vi "ConfigDevice.vi"(8 "error in (no error)":errorcluster, 11 "NhRegenGridSim in":refnum<class "NHRGridSim.lvclass">) -> (0 "error out":errorcluster, 3 "NhRegenGridSim out":refnum<class "NHRGridSim.lvclass">)   [LabVIEW 2018, in "AcPwrPlugins.lvlib" / "NHRGridSim.lvclass"]
doc: "This VI configures the instrument for the properties set such as instrument mode, slew, power level, etc."
uses:
  NHRGridSim.lvclass
  TypeDefs/ConfigDevicesTypeDef.ctl
  <instrlib>/NH Research 9400 Series/Public/Utility/Query Capabilities (Aperture).vi
  <vilib>/Utility/error.llb/Error Cluster From Error Code.vi
  <vilib>/ErrorRing/Error Ring.xnode
  <instrlib>/NH Research 9400 Series/NH Research 9400 Series.lvlib
  TypeDefs/RangeCheck.ctl
  <instrlib>/NH Research 9400 Series/Public/Configure/Configure Setpoint (Frequency).vi
  <instrlib>/NH Research 9400 Series/Public/Configure/Configure Range (Voltage).vi
  <instrlib>/NH Research 9400 Series/Public/Configure/Configure Range (Current).vi
  <instrlib>/NH Research 9400 Series/Public/Configure/Configure Slew Rate (Voltage).vi
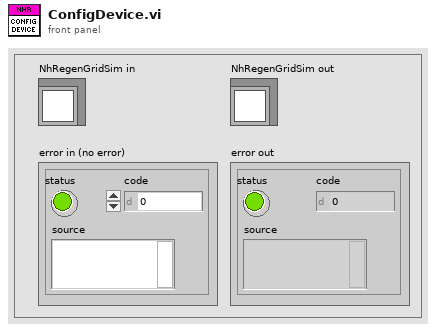
[diagram p1: front panel]
types:
  T1 = typedef "AcPwrPlugins.lvlib/NHRGridSim.lvclass/ConfigDevicesTypeDef.ctl" = enum16{"SelectMode", "SelectInstrument", "Safety", "WatchDog", "SlewRate", "RegulationGain", "Range", "Frequency", "Synchronization", "Measurement"}
  T2 = typedef "AcPwrPlugins.lvlib/NHRGridSim.lvclass/NHRGrid_Device(s)Settings.ctl" = cluster{"MeasName":string, "Hardware":T3}
  T3 = typedef "AcPwrPlugins.lvlib/NHRGridSim.lvclass/NHRGrid_Hardware.ctl" = cluster{"Handle":string, "Reset":bool, "Mode":T4, "ID Query":bool, "Logical Instrument":T5, "Connected":bool}
  T4 = typedef "AcPwrPlugins.lvlib/NHRGridSim.lvclass/NHRGrid_Modes.ctl" = u8
  T5 = typedef "AcPwrPlugins.lvlib/NHRGridSim.lvclass/NHRGrid_Logical_Instrument.ctl" = cluster{"Name":string, "Vout (V)":dbl, "I limit (A)":dbl, "P limit (W)":dbl, "FreqOut (Hz)":dbl, "Ranges":cluster{"Voltage (V)":u16, "Current (A)":u16}, "Configure Instrument":u16, "Aperture (cycles)":i32, "AC Wave Shape":u16, "VType":string, "IType":string, "Phases":T6, "Slew Rates":T7, "Safety Trips":T8}[]
  T6 = typedef "AcPwrPlugins.lvlib/NHRGridSim.lvclass/NHRGrid_Phases.ctl" = cluster{"A-Volts (V)":dbl, "B-Volts (V)":dbl, "C-Volts (V)":dbl, "A-Curr (A)":dbl, "B-Curr (A)":dbl, "C-Curr (A)":dbl, "A-Power (W)":dbl, "B-Power (W)":dbl, "C-Power (W)":dbl, "Change at (Deg)":dbl, "B-Angle (Deg)":dbl, "C-Angle (Deg)":dbl}
  T7 = typedef "AcPwrPlugins.lvlib/NHRGridSim.lvclass/NHRGrid_SlewRates.ctl" = cluster{"Vmax (V/s)":dbl, "Vmin (V/s)":dbl, "Imax (A/s)":dbl, "Imin (A/s)":dbl, "Pmax (W/s)":dbl, "Pmin (W/s)":dbl, "Freq Max (Hz/s)":dbl, "Freq Min (Hz/s)":dbl, "Phase Angle Max (Deg/s)":dbl, "Phase Angle Min (Deg/s)":dbl}
  T8 = typedef "AcPwrPlugins.lvlib/NHRGridSim.lvclass/NHRGrid_SafetyTrips.ctl" = cluster{"Vmax (V)":dbl, "Vmin (V)":dbl, "Vmax Time (s)":dbl, "Vmin Time (s)":dbl, "Imax Source (A)":dbl, "Imax Sink (A)":dbl, "Imax Source Time (s)":dbl, "Imax Sink Time (s)":dbl, "Pmax Source (W)":dbl, "Pmax Sink (W)":dbl, "Pmax Source Time (s)":dbl, "Pmax Sink Time (s)":dbl, "Absolute Volt Peak":dbl, "Enable Volt Peak":bool, "Absolute Curr Peak":dbl, "Enable Curr Peak":bool}
  T9 = typedef "AcPwrPlugins.lvlib/NHRGridSim.lvclass/RangeCheck.ctl" = enum16{"ApertureLength", "NumberOfSamples", "SlewAngleMultiPhaseAB", "SlewAngleMultiPhaseAC", "RegulationGain", "VoltageRange", "CurrentRange", "PhaseAngle", "Power", "Current", "Voltage", "Frequency"}[]
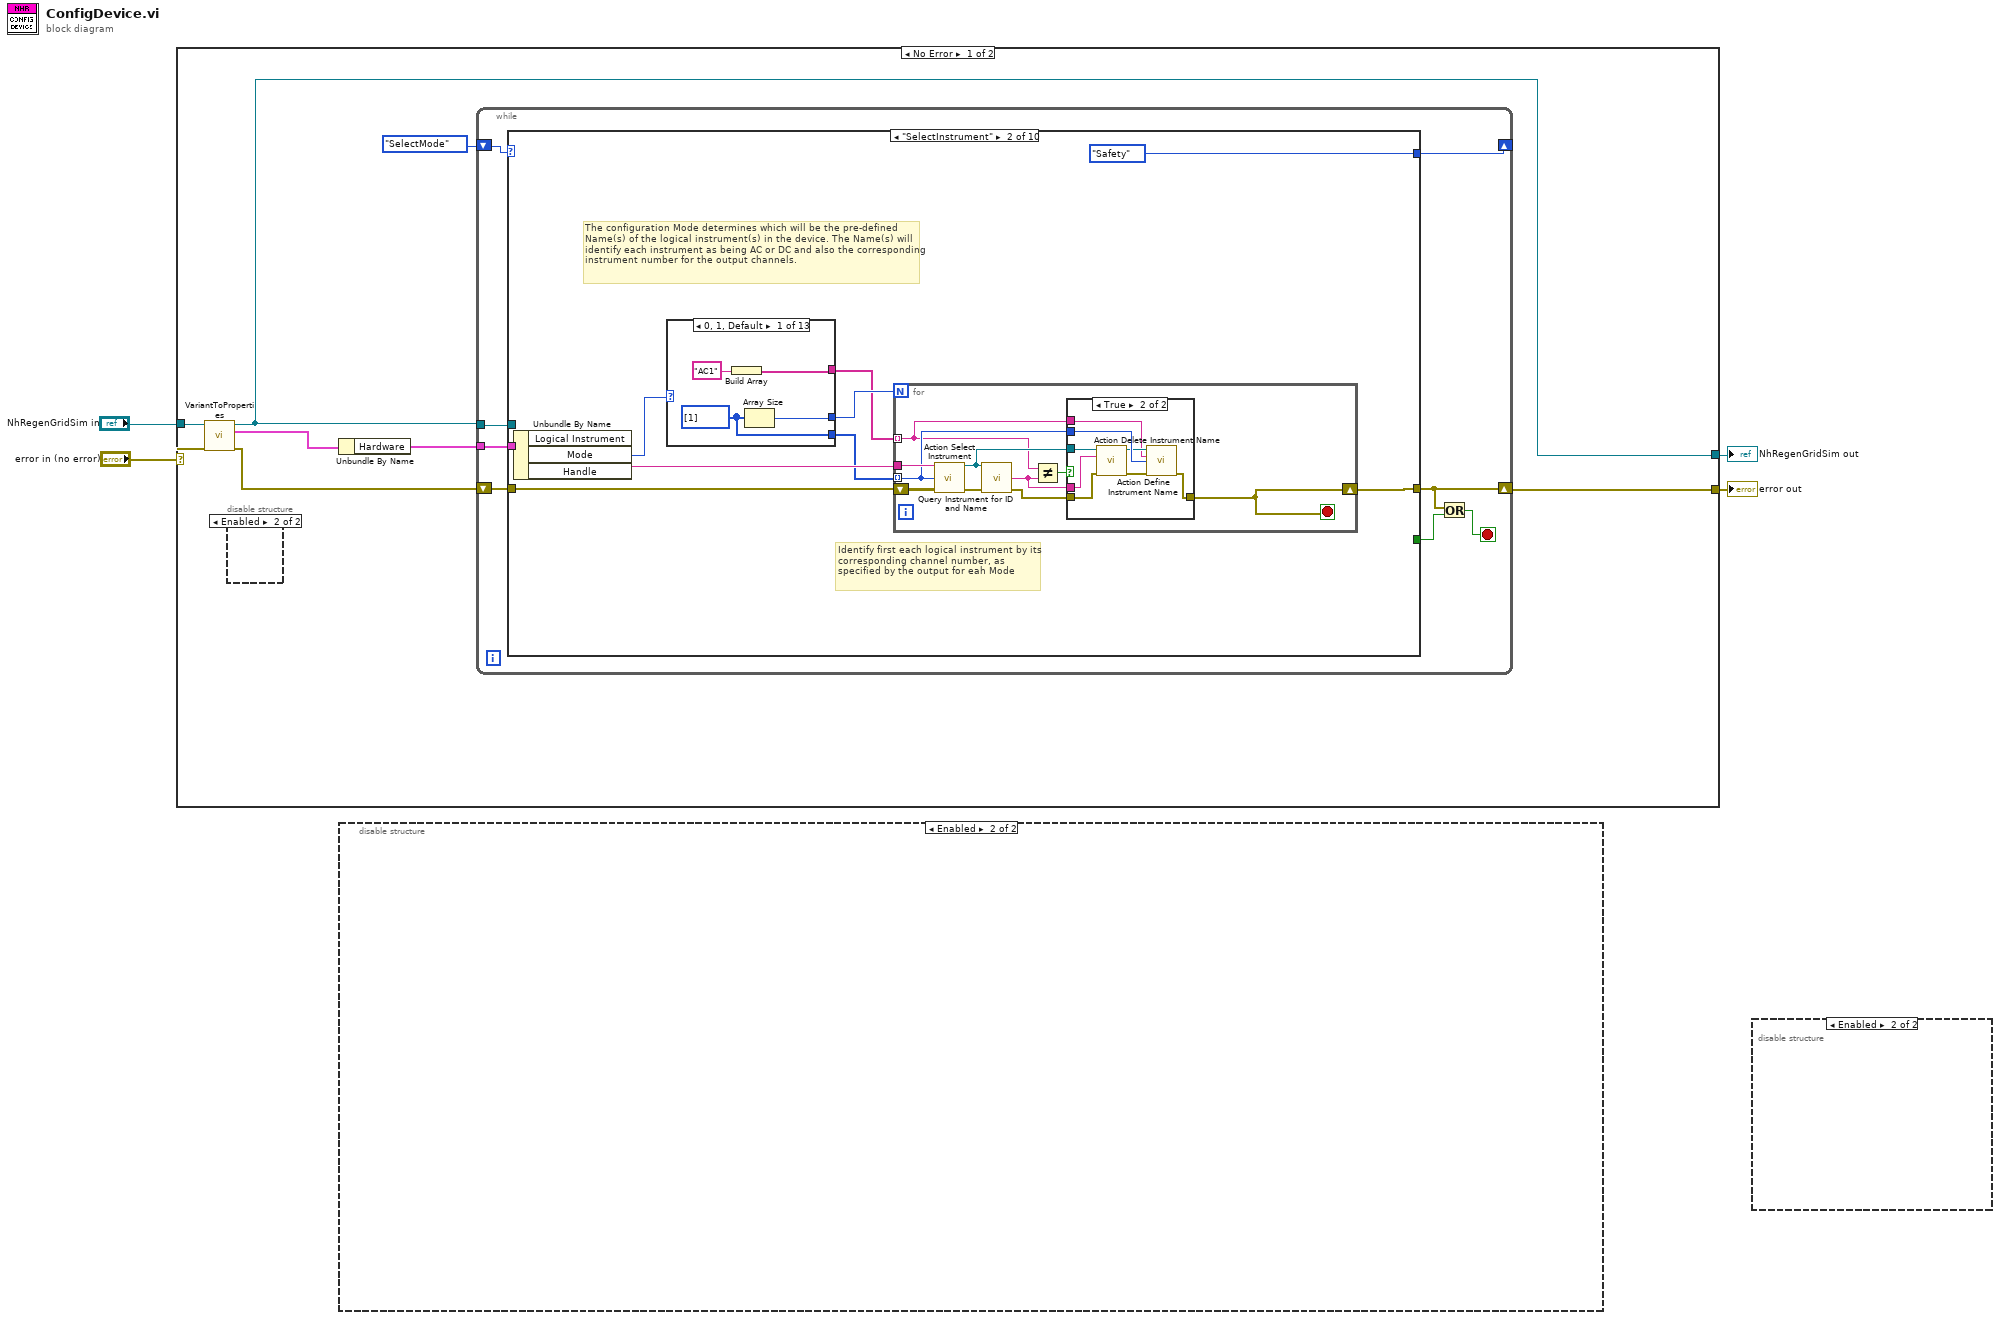
[diagram p0: block diagram]
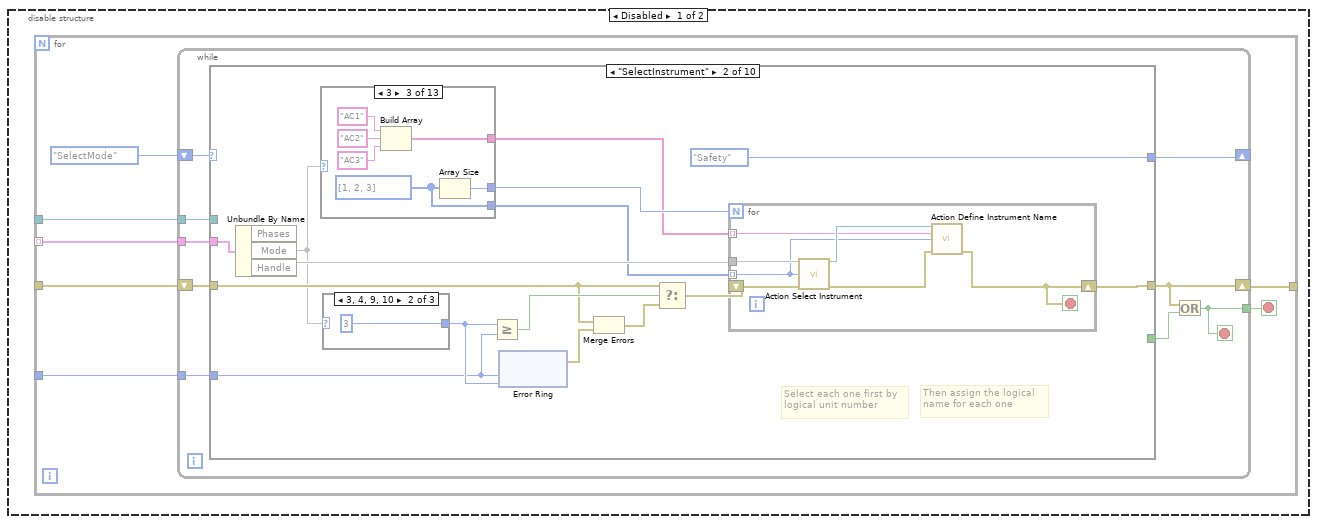
[diagram p2: hidden frame]
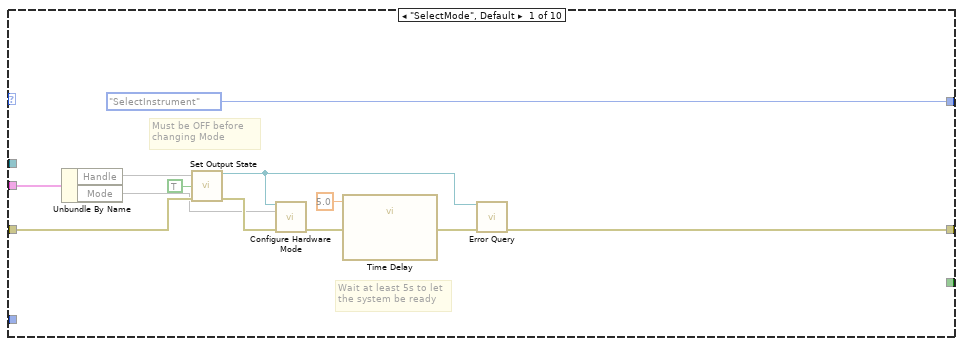
[diagram p3: hidden frame]
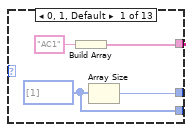
[diagram p4: hidden frame]
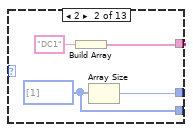
[diagram p5: hidden frame]
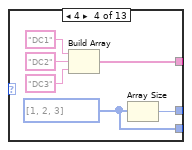
[diagram p6: hidden frame]
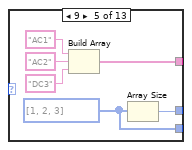
[diagram p7: hidden frame]
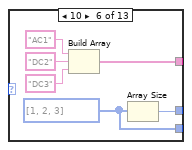
[diagram p8: hidden frame]
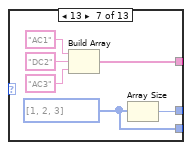
[diagram p9: hidden frame]
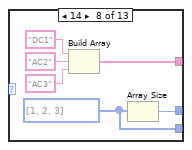
[diagram p10: hidden frame]
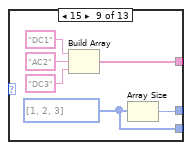
[diagram p11: hidden frame]
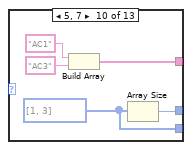
[diagram p12: hidden frame]
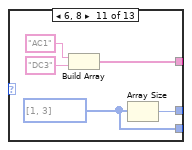
[diagram p13: hidden frame]
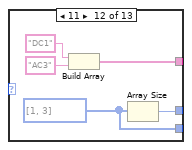
[diagram p14: hidden frame]
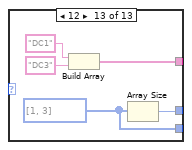
[diagram p15: hidden frame]
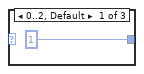
[diagram p16: hidden frame]
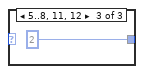
[diagram p17: hidden frame]
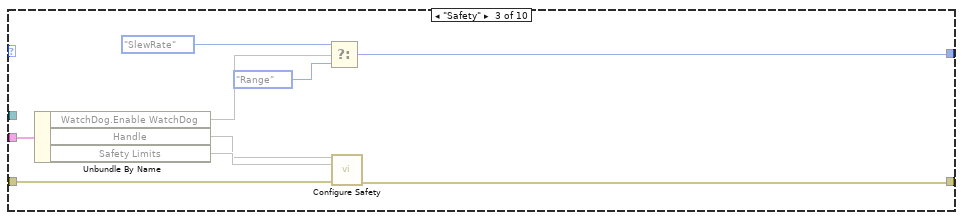
[diagram p18: hidden frame]
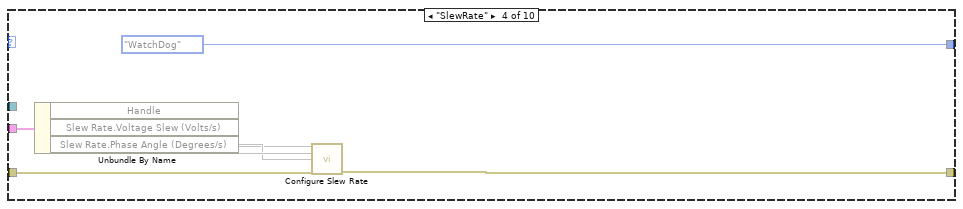
[diagram p19: hidden frame]
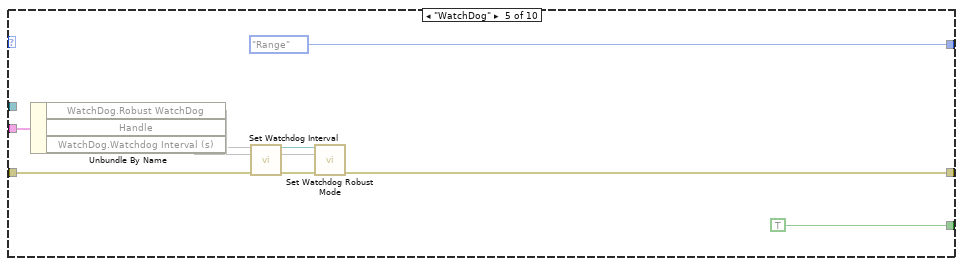
[diagram p20: hidden frame]
diagram:
  n1 = case shown="No Error" "error in (no error)" {
    selector: "error in (no error)" -> [w12 w267]
    tunnel: "NhRegenGridSim in" -> [w11 w268]
    tunnel: [w5 w268] -> w2
    tunnel: [w10 w267] -> w1
    frame No Error {
      n2 = call "VariantToProperties.vi"("NHRGridSim in"=w11, "error in (no error)"=w12) -> ("NHRGridSim out"=w5:refnum<class "NHRGridSim.lvclass">, "Device(s)Settings"=w7:T2, "error out"=w6:errorcluster)  [unwired: 8 in, 3 out]
      n3 = disable-structure shown="Enabled" {
        frame Disabled {
          n4 = call "CheckNumberOfPhases.vi"() -> ()  [unwired: 8 in, 4 out]
        }
        frame Enabled {
        }
      }
      n5 = Unbundle By Name(w7) -> ("Hardware"=w8:T3)
      n6 = while {
        shift-right: [w18] -> _
        shift-left: ConfigDevicesTypeDef."SelectMode" ("AcPwrPlugins.lvlib:NhRegenGridSim.lvclass:ConfigDevicesTypeDef") -> [w16]
        tunnel: w8 -> [w19]
        tunnel: w5 -> [w20]
        shift-right: [w14] -> w10
        shift-left: w6 -> [w17]
        stop <- w13 stop-if-true
        n7 = case shown="\"SelectInstrument\"" w16 {
          selector: w16 -> [_ _ _ _ _ _ _ _ _ w231]
          tunnel: w20 -> [_ _ _ _ _ w170 w186 w203 _ w227]
          tunnel: w19 -> [w31 w40 w133 w147 w155 w172 w188 w205 w218 w230]
          tunnel: [ConfigDevicesTypeDef."SelectInstrument" ("AcPwrPlugins.lvlib:NhRegenGridSim.lvclass:ConfigDevicesTypeDef") ConfigDevicesTypeDef."Safety" ("AcPwrPlugins.lvlib:NhRegenGridSim.lvclass:ConfigDevicesTypeDef") w130 ConfigDevicesTypeDef."WatchDog" ("AcPwrPlugins.lvlib:NhRegenGridSim.lvclass:ConfigDevicesTypeDef") ConfigDevicesTypeDef."Range" ("AcPwrPlugins.lvlib:NhRegenGridSim.lvclass:ConfigDevicesTypeDef") ConfigDevicesTypeDef."Range" ("AcPwrPlugins.lvlib:NhRegenGridSim.lvclass:ConfigDevicesTypeDef") ConfigDevicesTypeDef."Frequency" ("AcPwrPlugins.lvlib:NhRegenGridSim.lvclass:ConfigDevicesTypeDef") ConfigDevicesTypeDef."Synchronization" ("AcPwrPlugins.lvlib:NhRegenGridSim.lvclass:ConfigDevicesTypeDef") ConfigDevicesTypeDef."Measurement" ("AcPwrPlugins.lvlib:NhRegenGridSim.lvclass:ConfigDevicesTypeDef") w231] -> w18
          tunnel: w17 -> [w26 w32 w132 w146 w158 w169 w187 w204 w217 w226]
          tunnel: [w21 w39 w131 w144 w157 w171 w184 w201 w215 w225] -> w14
          tunnel: [_ _ _ _ TRUE TRUE _ _ _ TRUE] -> w15
          frame "SelectMode", Default {
            # "Set the desired MODE for the device. This will determine how many logical instruments will be configured, and which type each (AC or DC)"
            # "Wait at least 5s to let the system be ready"
            # "Must disable ALL outputs for all instruments before making any new settings"
            n8 = Unbundle By Name(w31) -> ("Handle"=w28:string, "Mode"=w25:T4)
            n9 = call <instrlib>:"Set Output State.vi"("VISA resource name"=w28, "All (F: Disable)"=TRUE, "error in (no error)"=w26) -> ("VISA resource name out"=w22:refnum<visa-resource-name>, "error out"=w27:errorcluster)  [unwired: 11 in]
            n10 = call <instrlib>:"Configure Hardware Mode.vi"("VISA resource name"=w22, "Mode"=w25, "error in (no error)"=w27) -> ("error out"=w24:errorcluster)  [unwired: 11 in, 1 out]
            n11 = call "Time Delay"("error in (no error)"=w24, "Delay Time (s)"=5.0) -> ("error out"=w21:errorcluster)  [unwired: 9 in]
          }
          frame "SelectInstrument" {
            # "The configuration Mode determines which will be the pre-defined Name(s) of the logical instrument(s) in the device. The Name(s) will identify each instrument as being AC or DC and also the corresponding instrument number for the output channels."
            # "Identify first each logical instrument by its corresponding channel number, as specified by the output for eah Mode"
            n12 = Unbundle By Name(w40) -> ("Mode"=w36:T4, "Handle"=w37:string)  [unwired: 1 out]
            n13 = case shown="0, 1, Default" w36 {
              tunnel: [w44 w48 w54 w60 w66 w72 w78 w84 w90 w95 w100 w105 w110] -> w35
              tunnel: [w43 w47 w53 w59 w65 w71 w77 w83 w89 w94 w99 w104 w109] -> w34
              tunnel: [w41 w45 w51 w57 w63 w69 w75 w81 w87 w92 w97 w102 w107] -> w33
              frame 0, 1, Default {
                w43 = u32[] [1]
                n14 = Build Array("AC1") -> (w41:string[])
                n15 = Array Size(array=w43) -> (size(s)=w44:i32)
              }
              frame 2 {
                w47 = u32[] [1]
                n16 = Build Array("DC1") -> (w45:string[])
                n17 = Array Size(array=w47) -> (size(s)=w48:i32)
              }
              frame 3 {
                w53 = u32[] [1, 2, 3]
                n18 = Build Array("AC1", "AC2", "AC3") -> (w51:string[])
                n19 = Array Size(array=w53) -> (size(s)=w54:i32)
              }
              frame 4 {
                w59 = u32[] [1, 2, 3]
                n20 = Build Array("DC1", "DC2", "DC3") -> (w57:string[])
                n21 = Array Size(array=w59) -> (size(s)=w60:i32)
              }
              frame 9 {
                w65 = u32[] [1, 2, 3]
                n22 = Build Array("AC1", "AC2", "DC3") -> (w63:string[])
                n23 = Array Size(array=w65) -> (size(s)=w66:i32)
              }
              frame 10 {
                w71 = u32[] [1, 2, 3]
                n24 = Build Array("AC1", "DC2", "DC3") -> (w69:string[])
                n25 = Array Size(array=w71) -> (size(s)=w72:i32)
              }
              frame 13 {
                w77 = u32[] [1, 2, 3]
                n26 = Build Array("AC1", "DC2", "AC3") -> (w75:string[])
                n27 = Array Size(array=w77) -> (size(s)=w78:i32)
              }
              frame 14 {
                w83 = u32[] [1, 2, 3]
                n28 = Build Array("DC1", "AC2", "AC3") -> (w81:string[])
                n29 = Array Size(array=w83) -> (size(s)=w84:i32)
              }
              frame 15 {
                w89 = u32[] [1, 2, 3]
                n30 = Build Array("DC1", "AC2", "DC3") -> (w87:string[])
                n31 = Array Size(array=w89) -> (size(s)=w90:i32)
              }
              frame 5, 7 {
                w94 = u32[] [1, 3]
                n32 = Build Array("AC1", "AC3") -> (w92:string[])
                n33 = Array Size(array=w94) -> (size(s)=w95:i32)
              }
              frame 6, 8 {
                w99 = u32[] [1, 3]
                n34 = Build Array("AC1", "DC3") -> (w97:string[])
                n35 = Array Size(array=w99) -> (size(s)=w100:i32)
              }
              frame 11 {
                w104 = u32[] [1, 3]
                n36 = Build Array("DC1", "AC3") -> (w102:string[])
                n37 = Array Size(array=w104) -> (size(s)=w105:i32)
              }
              frame 12 {
                w109 = u32[] [1, 3]
                n38 = Build Array("DC1", "DC3") -> (w107:string[])
                n39 = Array Size(array=w109) -> (size(s)=w110:i32)
              }
            }
            n40 = for {
              N: w35 -> [_]
              shift-right: [w111] -> w39
              shift-left: w32 -> [w120]
              tunnel: w37 -> [w119]
              tunnel: w33 -> [w112] mode=indexing
              tunnel: w34 -> [w116] mode=indexing
              stop <- w111 stop-if-true
              n41 = call <instrlib>:"Action Select Instrument.vi"("VISA resource name"=w119, "Logical Instrument Number"=w116, "error in (no error)"=w120) -> ("VISA resource name out"=w115:refnum<visa-resource-name>, "error out"=w118:errorcluster)  [unwired: 11 in]
              n42 = call <instrlib>:"Query Instrument for ID and Name.vi"("VISA resource name"=w115, "error in (no error)"=w118) -> ("Logical Instrument Name"=w114:string, "error out"=w113:errorcluster)  [unwired: 10 in, 2 out]
              n43 = Not Equal?(x=w112, y=w114) -> (x != y?=w117:bool)
              n44 = case shown="True" w117 {
                tunnel: w116 -> [_ w129]
                tunnel: w115 -> [_ w128]
                tunnel: w114 -> [_ w126]
                tunnel: w113 -> [w121 w125]
                tunnel: w112 -> [_ w123]
                tunnel: [w121 w122] -> w111
                frame False {
                }
                frame True {
                  n45 = call <instrlib>:"Action Delete Instrument Name.vi"("VISA resource name"=w128, "Logical Instrument Name"=w126, "error in (no error)"=w125) -> ("VISA resource name out"=w127:refnum<visa-resource-name>, "error out"=w124:errorcluster)  [unwired: 11 in]
                  n46 = call <instrlib>:"Action Define Instrument Name.vi"("VISA resource name"=w127, "Logical Instrument Name"=w123, "Logical Instrument Number"=w129, "error in (no error)"=w124) -> ("error out"=w122:errorcluster)  [unwired: 10 in, 1 out]
                }
              }
            }
          }
          frame "Safety" {
            n47 = disable-structure shown="Enabled" {
              disable-tunnel: w133 -> [w142 _]
              disable-tunnel: w132 -> [w141 w143]
              disable-tunnel: [w140 w143] -> w131
              disable-tunnel: [w137 _] -> w130
              frame Disabled {
                n48 = Unbundle By Name(w142) -> ("Enable WatchDog"=w139, "Handle"=w134:string, "Safety Limits"=w135)
                n49 = Select(t=ConfigDevicesTypeDef."SlewRate" ("AcPwrPlugins.lvlib:NhRegenGridSim.lvclass:ConfigDevicesTypeDef"), s=w139, f=ConfigDevicesTypeDef."Range" ("AcPwrPlugins.lvlib:NhRegenGridSim.lvclass:ConfigDevicesTypeDef")) -> (s? t:f=w137:T1)
                n50 = call <instrlib>:"Configure Safety.vi"("VISA resource name"=w134, "Safety Limits"=w135, "error in (no error)"=w141) -> ("error out"=w140:errorcluster)  [unwired: 11 in, 1 out]
              }
              frame Enabled {
              }
            }
          }
          frame "SlewRate" {
            n51 = disable-structure shown="Enabled" {
              disable-tunnel: w147 -> [w153 _]
              disable-tunnel: w146 -> [w152 w154]
              disable-tunnel: [w151 w154] -> w144
              frame Disabled {
                n52 = Unbundle By Name(w153) -> ("Handle"=w148:string, "Voltage Slew (Volts/s)"=w150, "Phase Angle (Degrees/s)"=w149)
                n53 = call-poly <instrlib>:"Configure Slew Rate.vi"("VISA resource name"=w148, "Voltage Slew Rate (0 V per sec)"=w150, 7:w149, "error in (no error)"=w152) -> ("error out"=w151:errorcluster)  [unwired: 10 in, 1 out]
              }
              frame Enabled {
              }
            }
          }
          frame "WatchDog" {
            n54 = disable-structure shown="Enabled" {
              disable-tunnel: w158 -> [w167 w168]
              disable-tunnel: [w164 w168] -> w157
              disable-tunnel: w155 -> [w163 _]
              frame Disabled {
                n55 = Unbundle By Name(w163) -> ("Robust WatchDog"=w162, "Handle"=w160:string, "Watchdog Interval (s)"=w161)
                n56 = call <instrlib>:"Set Watchdog Interval.vi"("VISA resource name"=w160, "Watchdog Interval (s)"=w161, "error in (no error)"=w167) -> ("VISA resource name out"=w165:refnum<visa-resource-name>, "error out"=w166:errorcluster)  [unwired: 11 in]
                n57 = call <instrlib>:"Set Watchdog Robust Mode.vi"("VISA resource name"=w165, "Robust Mode (F: Disable)"=w162, "error in (no error)"=w166) -> ("error out"=w164:errorcluster)  [unwired: 11 in, 1 out]
              }
              frame Enabled {
              }
            }
          }
          frame "RegulationGain" {
            n58 = disable-structure shown="Enabled" {
              disable-tunnel: w172 -> [w182 _]
              disable-tunnel: [w181 w183] -> w171
              disable-tunnel: w170 -> [w180 _]
              disable-tunnel: w169 -> [w179 w183]
              frame Disabled {
                w177 = T9 [enum."RegulationGain"] items=["ApertureLength", "NumberOfSamples", "SlewAngleMultiPhaseAB", "SlewAngleMultiPhaseAC", "RegulationGain", "VoltageRange", "CurrentRange", "PhaseAngle", "Power", "Current", "Voltage", "Frequency"] ("RangeCheck")
                n59 = Unbundle By Name(w182) -> ("Handle"=w176:string, "Regulation Gain"=w175)
                n60 = call-dynamic "RangeCheck.vi"("NhRegenGridSim in"=w180, "RangeCheck"=w177, "error in (no error)"=w179) -> ("error out"=w178:errorcluster)  [unwired: 6 in, 1 out]
                n61 = call <instrlib>:"Configure Regulation Gain.vi"("VISA resource name"=w176, "Regulation Gain (0)"=w175, "error in (no error)"=w178) -> ("error out"=w181:errorcluster)  [unwired: 11 in, 1 out]
              }
              frame Enabled {
              }
            }
          }
          frame "Range" {
            n62 = disable-structure shown="Enabled" {
              disable-tunnel: w188 -> [w197 _]
              disable-tunnel: w187 -> [w195 w200]
              disable-tunnel: w186 -> [w193 _]
              disable-tunnel: [w192 w200] -> w184
              frame Disabled {
                w191 = T9 [enum."Voltage", enum."Current"] items=["ApertureLength", "NumberOfSamples", "SlewAngleMultiPhaseAB", "SlewAngleMultiPhaseAC", "RegulationGain", "VoltageRange", "CurrentRange", "PhaseAngle", "Power", "Current", "Voltage", "Frequency"] ("RangeCheck")
                n63 = Unbundle By Name(w197) -> ("Irange (A)"=w196, "Handle"=w190:string, "Vrange (V)"=w189)
                n64 = call-dynamic "RangeCheck.vi"("NhRegenGridSim in"=w193, "RangeCheck"=w191, "error in (no error)"=w195) -> ("error out"=w194:errorcluster)  [unwired: 6 in, 1 out]
                n65 = call-poly <instrlib>:"Configure Range.vi"("VISA resource name"=w190, "Voltage Range (0 V)"=w189, "error in (no error)"=w194) -> ("VISA resource name out"=w198:refnum<visa-resource-name>, "error out"=w199:errorcluster)  [unwired: 11 in]
                n66 = call-poly <instrlib>:"Configure Range.vi"("VISA resource name"=w198, "Current Range (0 A)"=w196, "error in (no error)"=w199) -> ("error out"=w192:errorcluster)  [unwired: 11 in, 1 out]
              }
              frame Enabled {
              }
            }
          }
          frame "Frequency" {
            n67 = disable-structure shown="Enabled" {
              disable-tunnel: w205 -> [w213 _]
              disable-tunnel: w204 -> [w211 w214]
              disable-tunnel: w203 -> [w210 _]
              disable-tunnel: [w209 w214] -> w201
              frame Disabled {
                w207 = T9 [enum."Frequency"] items=["ApertureLength", "NumberOfSamples", "SlewAngleMultiPhaseAB", "SlewAngleMultiPhaseAC", "RegulationGain", "VoltageRange", "CurrentRange", "PhaseAngle", "Power", "Current", "Voltage", "Frequency"] ("RangeCheck")
                n68 = Unbundle By Name(w213) -> ("Handle"=w206:string, "FreqOut (Hz)"=w212)
                n69 = call-dynamic "RangeCheck.vi"("NhRegenGridSim in"=w210, "RangeCheck"=w207, "error in (no error)"=w211) -> ("error out"=w208:errorcluster)  [unwired: 6 in, 1 out]
                n70 = call-poly <instrlib>:"Configure Setpoint.vi"("VISA resource name"=w206, "Output Frequency (60 Hz)"=w212, "error in (no error)"=w208) -> ("error out"=w209:errorcluster)  [unwired: 11 in, 1 out]
              }
              frame Enabled {
              }
            }
          }
          frame "Synchronization" {
            n71 = disable-structure shown="Disabled" {
              disable-tunnel: w218 -> [w223 _]
              disable-tunnel: w217 -> [w222 w224]
              disable-tunnel: [w221 w224] -> w215
              frame Disabled {
                n72 = Unbundle By Name(w223) -> ("Handle"=w219:string, "Synchronize Output \nto Phase"=w220)
                n73 = call <instrlib>:"Configure Synchronization.vi"("VISA resource name"=w219, "Synchronization (F: Off)"=w220, "error in (no error)"=w222) -> ("error out"=w221:errorcluster)  [unwired: 11 in, 1 out]
              }
              frame Enabled {
              }
            }
          }
          frame "Measurement" {
            n74 = Unbundle By Name(w230) -> ("Handle"=w228:string, "Logical Instrument"=w229:T5)
            n75 = for {
              tunnel: w229 -> [w244] mode=indexing
              tunnel: w228 -> [w242]
              tunnel: w227 -> [_]
              shift-right: [w238] -> w225
              shift-left: w226 -> [w239]
              # "Change to seconds"
              n76 = Unbundle By Name(w244) -> ("Aperture (cycles)"=w241:i32)
              n77 = call-poly <instrlib>:"Query Capabilities.vi"("VISA resource name"=w242, "error in (no error)"=w239) -> ("VISA resource name out"=w243:refnum<visa-resource-name>, "Aperture Min (s)"=w234:dbl, "Aperture Max (s)"=w233:dbl, "error out"=w237:errorcluster)  [unwired: 10 in]
              n78 = Divide(x=w241, y=60.0) -> (x/y=w235:dbl)
              n79 = In Range and Coerce(upper limit=w233, x=w235, lower limit=w234) -> (In Range?=w236:bool)  [unwired: 1 out]
              n80 = case shown="False" w236 {
                selector: w236 -> [w245 _]
                tunnel: w243 -> [_ w266]
                tunnel: [w252 w265] -> w238
                tunnel: w237 -> [w247 w264]
                tunnel: w235 -> [w246 w263]
                tunnel: w234 -> [w249 _]
                tunnel: w233 -> [w248 _]
                frame False {
                  n81 = xnode "Error Ring"("parameter 0"="ApertureLength", "parameter 1"=w246, "parameter 2"=w249, "parameter 3"=w248) -> ("error out"=w251:errorcluster)
                  n82 = Select(t=w247, s=w245, f=w251) -> (s? t:f=w252:errorcluster)
                }
                frame True {
                  n83 = call <instrlib>:"Set Aperture Length.vi"("VISA resource name"=w266, "Aperture Length (s)"=w263, "error in (no error)"=w264) -> ("error out"=w265:errorcluster)  [unwired: 11 in, 1 out]
                }
              }
              n84 = disable-structure shown="Disabled" {
                frame Disabled {
                  n85 = call <instrlib>:"Set Number of Samples.vi"() -> ()  [unwired: 14 in, 2 out]
                }
                frame Enabled {
                }
              }
            }
          }
        }
        n86 = Or(x=w14, y=w15) -> (x .or. y?=w13:bool)
      }
    }
    frame Error {
    }
  }
  "NhRegenGridSim out" <- w2
  "error out" <- w1
  n87 = disable-structure shown="Enabled" {
    frame Disabled {
      n88 = for {
        tunnel: _ -> [w271] mode=indexing
        tunnel: _ -> [w275]
        tunnel: _ -> [w274]
        tunnel: [w273] -> _
        tunnel: _ -> [w269]
        stop <- w272 stop-if-true
        n89 = while {
          shift-right: [w282] -> _
          shift-left: ConfigDevicesTypeDef."SelectMode" ("AcPwrPlugins.lvlib:NhRegenGridSim.lvclass:ConfigDevicesTypeDef") -> [w280]
          tunnel: w271 -> [w283]
          tunnel: w275 -> [w284]
          shift-right: [w277] -> w273
          shift-left: w274 -> [w281]
          tunnel: [w276] -> w272
          tunnel: w269 -> [w279]
          stop <- w276 stop-if-true
          n90 = case shown="\"SelectInstrument\"" w280 {
            selector: w280 -> [_ _ _ _ _ _ _ _ _ w465]
            tunnel: w284 -> [_ _ _ _ _ w431 w441 w453 _ w471]
            tunnel: w283 -> [w296 w311 w408 w415 w419 w433 w445 w456 w462 w474]
            tunnel: [ConfigDevicesTypeDef."SelectInstrument" ("AcPwrPlugins.lvlib:NhRegenGridSim.lvclass:ConfigDevicesTypeDef") ConfigDevicesTypeDef."Safety" ("AcPwrPlugins.lvlib:NhRegenGridSim.lvclass:ConfigDevicesTypeDef") w403 ConfigDevicesTypeDef."WatchDog" ("AcPwrPlugins.lvlib:NhRegenGridSim.lvclass:ConfigDevicesTypeDef") ConfigDevicesTypeDef."Range" ("AcPwrPlugins.lvlib:NhRegenGridSim.lvclass:ConfigDevicesTypeDef") ConfigDevicesTypeDef."Range" ("AcPwrPlugins.lvlib:NhRegenGridSim.lvclass:ConfigDevicesTypeDef") ConfigDevicesTypeDef."Frequency" ("AcPwrPlugins.lvlib:NhRegenGridSim.lvclass:ConfigDevicesTypeDef") ConfigDevicesTypeDef."Synchronization" ("AcPwrPlugins.lvlib:NhRegenGridSim.lvclass:ConfigDevicesTypeDef") ConfigDevicesTypeDef."Measurement" ("AcPwrPlugins.lvlib:NhRegenGridSim.lvclass:ConfigDevicesTypeDef") w465] -> w282
            tunnel: w281 -> [w291 w302 w407 w414 w424 w430 w443 w454 w461 w469]
            tunnel: [w289 w305 w406 w412 w421 w432 w439 w451 w459 w466] -> w277
            tunnel: [_ _ _ _ TRUE TRUE _ _ _ TRUE] -> w278
            tunnel: w279 -> [_ w304 _ _ _ _ _ _ _ _]
            frame "SelectMode", Default {
              # "Wait at least 5s to let the system be ready"
              # "Must be OFF before changing Mode"
              n91 = Unbundle By Name(w296) -> ("Handle"=w293, "Mode"=w290)
              n92 = call <instrlib>:"Set Output State.vi"("VISA resource name"=w293, "All (F: Disable)"=TRUE, "error in (no error)"=w291) -> ("VISA resource name out"=w285:refnum<visa-resource-name>, "error out"=w292:errorcluster)  [unwired: 11 in]
              n93 = call <instrlib>:"Configure Hardware Mode.vi"("VISA resource name"=w285, "Mode"=w290, "error in (no error)"=w292) -> ("error out"=w288:errorcluster)  [unwired: 11 in, 1 out]
              n94 = call "Time Delay"("error in (no error)"=w288, "Delay Time (s)"=5.0) -> ("error out"=w287:errorcluster)  [unwired: 9 in]
              n95 = call <instrlib>:"Error Query.vi"("VISA resource name"=w285, "error in (no error)"=w287) -> ("error out"=w289:errorcluster)  [unwired: 10 in, 3 out]
            }
            frame "SelectInstrument" {
              # "Then assign the logical name for each one"
              # "Select each one first by logical unit number"
              n96 = Unbundle By Name(w311) -> ("Mode"=w300, "Handle"=w301)  [unwired: 1 out]
              n97 = case shown="3" w300 {
                tunnel: [w315 w319 w325 w331 w337 w343 w349 w355 w361 w366 w371 w376 w381] -> w299
                tunnel: [w314 w318 w324 w330 w336 w342 w348 w354 w360 w365 w370 w375 w380] -> w298
                tunnel: [w312 w316 w322 w328 w334 w340 w346 w352 w358 w363 w368 w373 w378] -> w297
                frame 0, 1, Default {
                  w314 = u32[] [1]
                  n98 = Build Array("AC1") -> (w312:string[])
                  n99 = Array Size(array=w314) -> (size(s)=w315:i32)
                }
                frame 2 {
                  w318 = u32[] [1]
                  n100 = Build Array("DC1") -> (w316:string[])
                  n101 = Array Size(array=w318) -> (size(s)=w319:i32)
                }
                frame 3 {
                  w324 = u32[] [1, 2, 3]
                  n102 = Build Array("AC1", "AC2", "AC3") -> (w322:string[])
                  n103 = Array Size(array=w324) -> (size(s)=w325:i32)
                }
                frame 4 {
                  w330 = u32[] [1, 2, 3]
                  n104 = Build Array("DC1", "DC2", "DC3") -> (w328:string[])
                  n105 = Array Size(array=w330) -> (size(s)=w331:i32)
                }
                frame 9 {
                  w336 = u32[] [1, 2, 3]
                  n106 = Build Array("AC1", "AC2", "DC3") -> (w334:string[])
                  n107 = Array Size(array=w336) -> (size(s)=w337:i32)
                }
                frame 10 {
                  w342 = u32[] [1, 2, 3]
                  n108 = Build Array("AC1", "DC2", "DC3") -> (w340:string[])
                  n109 = Array Size(array=w342) -> (size(s)=w343:i32)
                }
                frame 13 {
                  w348 = u32[] [1, 2, 3]
                  n110 = Build Array("AC1", "DC2", "AC3") -> (w346:string[])
                  n111 = Array Size(array=w348) -> (size(s)=w349:i32)
                }
                frame 14 {
                  w354 = u32[] [1, 2, 3]
                  n112 = Build Array("DC1", "AC2", "AC3") -> (w352:string[])
                  n113 = Array Size(array=w354) -> (size(s)=w355:i32)
                }
                frame 15 {
                  w360 = u32[] [1, 2, 3]
                  n114 = Build Array("DC1", "AC2", "DC3") -> (w358:string[])
                  n115 = Array Size(array=w360) -> (size(s)=w361:i32)
                }
                frame 5, 7 {
                  w365 = u32[] [1, 3]
                  n116 = Build Array("AC1", "AC3") -> (w363:string[])
                  n117 = Array Size(array=w365) -> (size(s)=w366:i32)
                }
                frame 6, 8 {
                  w370 = u32[] [1, 3]
                  n118 = Build Array("AC1", "DC3") -> (w368:string[])
                  n119 = Array Size(array=w370) -> (size(s)=w371:i32)
                }
                frame 11 {
                  w375 = u32[] [1, 3]
                  n120 = Build Array("DC1", "AC3") -> (w373:string[])
                  n121 = Array Size(array=w375) -> (size(s)=w376:i32)
                }
                frame 12 {
                  w380 = u32[] [1, 3]
                  n122 = Build Array("DC1", "DC3") -> (w378:string[])
                  n123 = Array Size(array=w380) -> (size(s)=w381:i32)
                }
              }
              n124 = case shown="3, 4, 9, 10" w300 {
                tunnel: [1 3 2] -> w307
                frame 0..2, Default {
                }
                frame 3, 4, 9, 10 {
                }
                frame 5..8, 11, 12 {
                }
              }
              n125 = Greater Or Equal?(x=w307, y=w304) -> (x >= y?=w310:bool)
              n126 = xnode "Error Ring"("parameter 0"=w304, "parameter 1"=w307) -> ("error out"=w306:errorcluster)
              n127 = Merge Errors(w302, w306) -> (w308:errorcluster)
              n128 = Select(t=w302, s=w310, f=w308) -> (s? t:f=w309:errorcluster)
              n129 = for {
                N: w299 -> [_]
                shift-right: [w396] -> w305
                shift-left: w309 -> [w399]
                tunnel: w301 -> [w398]
                tunnel: w297 -> [w394] mode=indexing
                tunnel: w298 -> [w393] mode=indexing
                stop <- w396 stop-if-true
                n130 = call <instrlib>:"Action Select Instrument.vi"("VISA resource name"=w398, "Logical Instrument Number"=w393, "error in (no error)"=w399) -> ("VISA resource name out"=w395:refnum<visa-resource-name>, "error out"=w397:errorcluster)  [unwired: 11 in]
                n131 = call <instrlib>:"Action Define Instrument Name.vi"("VISA resource name"=w395, "Logical Instrument Name"=w394, "Logical Instrument Number"=w393, "error in (no error)"=w397) -> ("error out"=w396:errorcluster)  [unwired: 10 in, 1 out]
              }
            }
            frame "Safety" {
              n132 = Unbundle By Name(w408) -> ("WatchDog.Enable WatchDog"=w405, "Handle"=w400, "Safety Limits"=w401)
              n133 = Select(t=ConfigDevicesTypeDef."SlewRate" ("AcPwrPlugins.lvlib:NhRegenGridSim.lvclass:ConfigDevicesTypeDef"), s=w405, f=ConfigDevicesTypeDef."Range" ("AcPwrPlugins.lvlib:NhRegenGridSim.lvclass:ConfigDevicesTypeDef")) -> (s? t:f=w403:T1)
              n134 = call <instrlib>:"Configure Safety.vi"("VISA resource name"=w400, "Safety Limits"=w401, "error in (no error)"=w407) -> ("error out"=w406:errorcluster)  [unwired: 11 in, 1 out]
            }
            frame "SlewRate" {
              n135 = Unbundle By Name(w415) -> ("Handle"=w409, "Slew Rate.Voltage Slew (Volts/s)"=w411, "Slew Rate.Phase Angle (Degrees/s)"=w410)
              n136 = call-poly <instrlib>:"Configure Slew Rate.vi"("VISA resource name"=w409, "Voltage Slew Rate (0 V per sec)"=w411, 7:w410, "error in (no error)"=w414) -> ("error out"=w412:errorcluster)  [unwired: 10 in, 1 out]
            }
            frame "WatchDog" {
              n137 = Unbundle By Name(w419) -> ("WatchDog.Robust WatchDog"=w418, "Handle"=w416, "WatchDog.Watchdog Interval (s)"=w417)
              n138 = call <instrlib>:"Set Watchdog Interval.vi"("VISA resource name"=w416, "Watchdog Interval (s)"=w417, "error in (no error)"=w424) -> ("VISA resource name out"=w422:refnum<visa-resource-name>, "error out"=w423:errorcluster)  [unwired: 11 in]
              n139 = call <instrlib>:"Set Watchdog Robust Mode.vi"("VISA resource name"=w422, "Robust Mode (F: Disable)"=w418, "error in (no error)"=w423) -> ("error out"=w421:errorcluster)  [unwired: 11 in, 1 out]
            }
            frame "RegulationGain" {
              w428 = T9 [enum."RegulationGain"] items=["ApertureLength", "NumberOfSamples", "SlewAngleMultiPhaseAB", "SlewAngleMultiPhaseAC", "RegulationGain", "VoltageRange", "CurrentRange", "PhaseAngle", "Power", "Current", "Voltage", "Frequency"] ("RangeCheck")
              n140 = Unbundle By Name(w433) -> ("Handle"=w427, "Regulation Gain"=w426)
              n141 = call-dynamic "RangeCheck.vi"("NhRegenGridSim in"=w431, "RangeCheck"=w428, "error in (no error)"=w430) -> ("error out"=w429:errorcluster)  [unwired: 6 in, 1 out]
              n142 = call <instrlib>:"Configure Regulation Gain.vi"("VISA resource name"=w427, "Regulation Gain (0)"=w426, "error in (no error)"=w429) -> ("error out"=w432:errorcluster)  [unwired: 11 in, 1 out]
            }
            frame "Range" {
              w438 = T9 [enum."Voltage", enum."Current"] items=["ApertureLength", "NumberOfSamples", "SlewAngleMultiPhaseAB", "SlewAngleMultiPhaseAC", "RegulationGain", "VoltageRange", "CurrentRange", "PhaseAngle", "Power", "Current", "Voltage", "Frequency"] ("RangeCheck")
              n143 = Unbundle By Name(w445) -> ("Ranges.Irange (A)"=w444, "Handle"=w437, "Ranges.Vrange (V)"=w436)
              n144 = call-dynamic "RangeCheck.vi"("NhRegenGridSim in"=w441, "RangeCheck"=w438, "error in (no error)"=w443) -> ("error out"=w442:errorcluster)  [unwired: 6 in, 1 out]
              n145 = call-poly <instrlib>:"Configure Range.vi"("VISA resource name"=w437, "Voltage Range (0 V)"=w436, "error in (no error)"=w442) -> ("VISA resource name out"=w446:refnum<visa-resource-name>, "error out"=w447:errorcluster)  [unwired: 11 in]
              n146 = call-poly <instrlib>:"Configure Range.vi"("VISA resource name"=w446, "Current Range (0 A)"=w444, "error in (no error)"=w447) -> ("error out"=w439:errorcluster)  [unwired: 11 in, 1 out]
            }
            frame "Frequency" {
              w449 = T9 [enum."Frequency"] items=["ApertureLength", "NumberOfSamples", "SlewAngleMultiPhaseAB", "SlewAngleMultiPhaseAC", "RegulationGain", "VoltageRange", "CurrentRange", "PhaseAngle", "Power", "Current", "Voltage", "Frequency"] ("RangeCheck")
              n147 = Unbundle By Name(w456) -> ("Handle"=w448, "FreqOut (Hz)"=w455)
              n148 = call-dynamic "RangeCheck.vi"("NhRegenGridSim in"=w453, "RangeCheck"=w449, "error in (no error)"=w454) -> ("error out"=w450:errorcluster)  [unwired: 6 in, 1 out]
              n149 = call-poly <instrlib>:"Configure Setpoint.vi"("VISA resource name"=w448, "Output Frequency (60 Hz)"=w455, "error in (no error)"=w450) -> ("error out"=w451:errorcluster)  [unwired: 11 in, 1 out]
            }
            frame "Synchronization" {
              n150 = Unbundle By Name(w462) -> ("Handle"=w457, "Synchronize Output \nto Phase"=w458)
              n151 = call <instrlib>:"Configure Synchronization.vi"("VISA resource name"=w457, "Synchronization (F: Off)"=w458, "error in (no error)"=w461) -> ("error out"=w459:errorcluster)  [unwired: 11 in, 1 out]
            }
            frame "Measurement" {
              w467 = T9 [enum."ApertureLength", enum."NumberOfSamples"] items=["ApertureLength", "NumberOfSamples", "SlewAngleMultiPhaseAB", "SlewAngleMultiPhaseAC", "RegulationGain", "VoltageRange", "CurrentRange", "PhaseAngle", "Power", "Current", "Voltage", "Frequency"] ("RangeCheck")
              n152 = Unbundle By Name(w474) -> ("Measurement.ApertureLength (s)"=w473, "Handle"=w463, "Measurement.NumberOfSamples"=w464)
              n153 = call-dynamic "RangeCheck.vi"("NhRegenGridSim in"=w471, "RangeCheck"=w467, "error in (no error)"=w469) -> ("error out"=w470:errorcluster)  [unwired: 6 in, 1 out]
              n154 = call <instrlib>:"Set Number of Samples.vi"("VISA resource name"=w463, "Number of Samples"=w464, "error in (no error)"=w470) -> ("VISA resource name out"=w472:refnum<visa-resource-name>, "error out"=w475:errorcluster)  [unwired: 11 in]
              n155 = call <instrlib>:"Set Aperture Length.vi"("VISA resource name"=w472, "Aperture Length (s)"=w473, "error in (no error)"=w475) -> ("error out"=w466:errorcluster)  [unwired: 11 in, 1 out]
            }
          }
          n156 = Or(x=w277, y=w278) -> (x .or. y?=w276:bool)
        }
      }
    }
    frame Enabled {
    }
  }
  n157 = disable-structure shown="Enabled" {
    frame Disabled {
      n158 = for {
        shift-right: [w479] -> _
        shift-left: _ -> [w483]
        tunnel: _ -> [w480]
        tunnel: _ -> [w482] mode=indexing
        i -> [w478]
        stop <- w479 stop-if-true
        n159 = Unbundle By Name(w482) -> ("Phase Name"=w481)
        n160 = Increment(x=w478) -> (x+1=w477:i32)
        n161 = To Unsigned Long Integer(number=w477) -> (unsigned 32bit integer=w476:u32)
        n162 = call <instrlib>:"Action Select Instrument.vi"("VISA resource name"=w480, "Logical Instrument Name"=w481, "Logical Instrument Number"=w476, "error in (no error)"=w483) -> ("error out"=w479:errorcluster)  [unwired: 10 in, 1 out]
      }
    }
    frame Enabled {
    }
  }
